vi "Set TempSP.vi"(8 "error in (no error)":errorcluster, 10 "Temp SP(C)":dbl, 11 "ThermPID in":refnum<class "ThermPID.lvclass">) -> (0 "error out":errorcluster, 3 "ThermPID out":refnum<class "ThermPID.lvclass">)   [LabVIEW 2023, in "ThermPID.lvclass"]
uses:
  ThermPID.lvclass
  ThermPID.lvclass/ThermPID.ctl
  PIDController/PIDController.lvclass
  <vilib>/NI/Modbus Library/API/Master/Modbus Master.lvclass
  PIDModBus/PIDModbus.lvlib
  PIDModBus/Controls/Register Enum.ctl
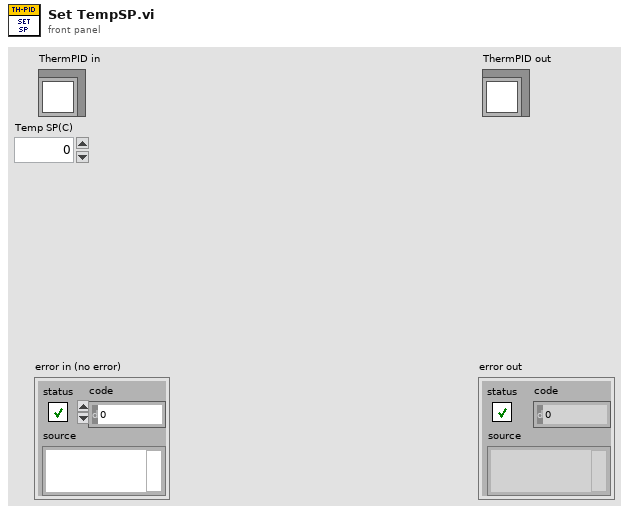
[diagram p1: front panel]
types:
  T1 = typedef "PIDModbus.lvlib/Register Enum.ctl" = u16
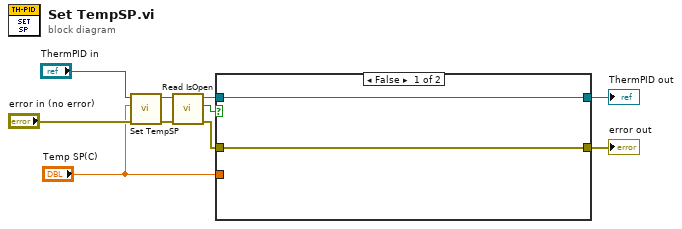
[diagram p0: block diagram]
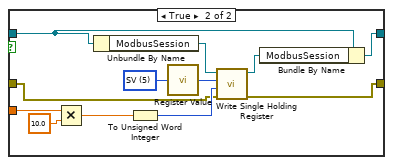
[diagram p2: hidden frame]
diagram:
  n1 = call-parent "Set TempSP.vi"("error in (no error)"="error in (no error)", "Temp SP(C)"="Temp SP(C)", "PIDController in"="ThermPID in") -> ("error out"=w4:errorcluster, "PIDController out"=w6:refnum<class "ThermPID.lvclass">)  [unwired: 7 in]
  n2 = call-dynamic "Read IsOpen.vi"("error in (no error)"=w4, "PIDController in"=w6) -> ("error out"=w3:errorcluster, "IsOpen"=w1:bool, "PIDController out"=w5:refnum<class "ThermPID.lvclass">)  [unwired: 7 in]
  n3 = case shown="False" w1 {
    tunnel: "Temp SP(C)" -> [_ w18]
    tunnel: [w11 w17] -> w7
    tunnel: w5 -> [w12 w16]
    tunnel: w3 -> [w11 w15]
    tunnel: [w12 w14] -> w2
    frame False {
    }
    frame True {
      w20 = T1 5 items=["PV"=0, "SV"=5, "P1"=24, "I1"=25, "D1"=26] ("Register")
      n4 = Multiply(x=w18, y=10.0) -> (x*y=w23:dbl)
      n5 = Unbundle By Name(w16) -> ("ModbusSession"=w19:refnum<class "Modbus Master.lvclass">)
      n6 = To Unsigned Word Integer(number=w23) -> (unsigned 16bit integer=w24:u16)
      n7 = call "Register Value.vi"("Register"=w20) -> ("RegAddr (Hex)"=w21:u16)
      n8 = call-dynamic "Write Single Holding Register.vi"("error in"=w15, "register to write"=w24, "address"=w21, "Modbus master in"=w19) -> ("error out"=w17:errorcluster, "Modbus master out"=w13:refnum<class "Modbus Master.lvclass">)  [unwired: 6 in]
      n9 = Bundle By Name(cluster=w16, "ModbusSession"=w13) -> (w14:refnum<class "ThermPID.lvclass">)
    }
  }
  "error out" <- w7
  "ThermPID out" <- w2
